vi "Get NumLevels From Flattened Object.vi"(1 "Flattened Object Data":u8[](array[numeric])) -> (0 "Number of Levels":u32)   [LabVIEW 2017, in "Composition.lvlib"]
doc: "Gets the number of class levels from flattened object data."
uses:
  Composition.lvlib
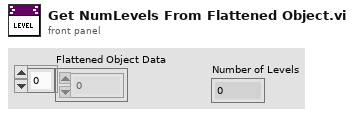
[diagram p1: front panel]
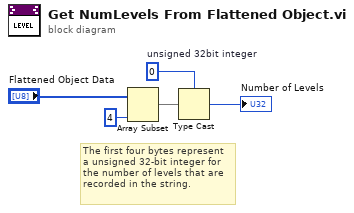
[diagram p0: block diagram]
diagram:
  w5 = u32 0  # unsigned 32bit integer
  # "The first four bytes represent\na unsigned 32-bit integer for\nthe number of levels that are\nrecorded in the string."
  n1 = Array Subset(array="Flattened Object Data", length=4 ("index")) -> (w4:u8[])  [unwired: 1 in]
  n2 = Type Cast(type=w5, x=w4) -> (*(type *) &x=→"Number of Levels":u32)
